vi "sender_info.vi"() -> ()   [LabVIEW 2016]
panel:
  in  "service_name":string
  in  "version":string
  in  "commit":string
  in  "package":string
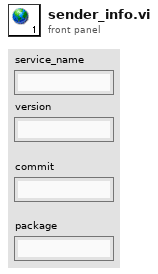
[diagram p1: front panel]
diagram:
